vi "Measure Line Distance (SubVI).vi"(9 "Input Valid?":bool=TRUE, 10 "X1 Y1":u32, 11 "X2 Y2":u32) -> (2 "Output Valid?":bool, 3 "Distance":u16)   [LabVIEW 2015]
uses:
  <vilib>/rvi/FXPMathLib/FxpSqrt/subVIs/nifxpmath_Sqrt_SimConfig.ctl
  <vilib>/fxp/LVFixedPointOverflowPolicyTypeDef.ctl
  <vilib>/rvi/FXPMathLib/FxpSqrt/simVIs/DllSqrtTemp_sub.vi
  <vilib>/rvi/FXPMathLib/FxpSub/XNode/nifxpmath_Sub.xnode
  <vilib>/rvi/FXPMathLib/FxpMul/XNode/nifxpmath_Multiplier.xnode
  <vilib>/rvi/FXPMathLib/FxpAdd/XNode/nifxpmath_Add.xnode
  <vilib>/rvi/FXPMathLib/FxpSqrt/XNode/nifxpmath_Sqrt.xnode
  <vilib>/rvi/FXPMathLib/sim/FxpSim.dll
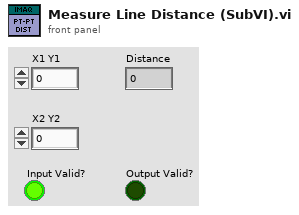
[diagram p1: front panel]
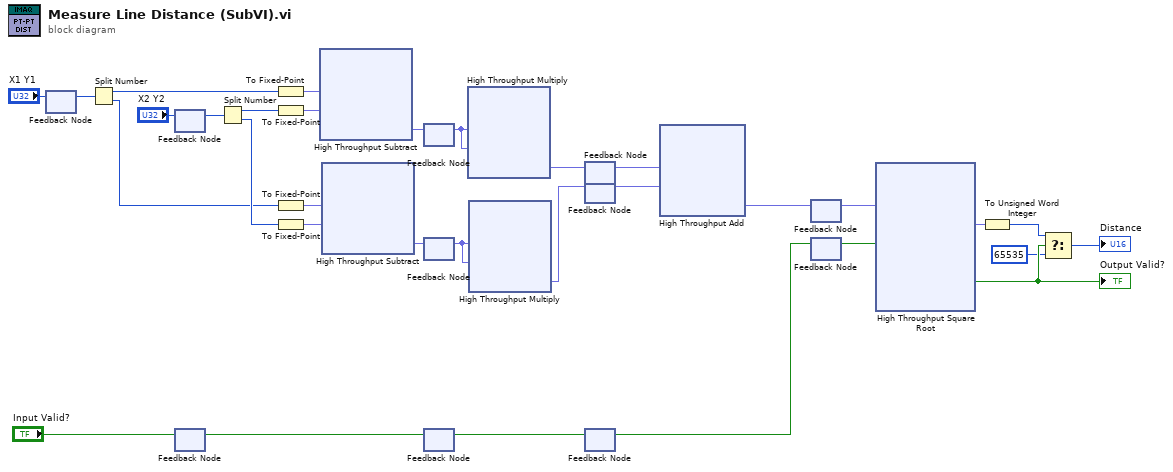
[diagram p0: block diagram]
diagram:
  n1 = feedback-in #1("X1 Y1") -> ()
  n2 = feedback #1() -> (w11:u32)  [unwired: 1 in]
  n3 = Split Number(x=w11) -> (hi(x)=w28:u16, lo(x)=w29:u16)
  n4 = feedback-in #2("X2 Y2") -> ()
  n5 = feedback #2() -> (w10:u32)  [unwired: 1 in]
  n6 = feedback-in #3("Input Valid?") -> ()
  n7 = feedback #3() -> (w9:bool)  [unwired: 1 in]
  n8 = Split Number(x=w10) -> (hi(x)=w31:u16, lo(x)=w32:u16)
  n9 = To Fixed-Point(number=w28) -> (fixed-point=w17:fxp<+/-,16,16>)  [unwired: 1 in]
  n10 = To Fixed-Point(number=w31) -> (fixed-point=w18:fxp<+/-,16,16>)  [unwired: 1 in]
  n11 = To Fixed-Point(number=w29) -> (fixed-point=w20:fxp<+/-,16,16>)  [unwired: 1 in]
  n12 = To Fixed-Point(number=w32) -> (fixed-point=w19:fxp<+/-,16,16>)  [unwired: 1 in]
  n13 = xnode "High Throughput Subtract"("x"=w17, "y"=w18) -> ("x-y"=w21:fxp<+/-,17,17>)
  n14 = xnode "High Throughput Subtract"("x"=w20, "y"=w19) -> ("x-y"=w22:fxp<+/-,17,17>)
  n15 = feedback-in #4(w21) -> ()
  n16 = feedback #4() -> (w8:fxp<+/-,17,17>)  [unwired: 1 in]
  n17 = feedback-in #5(w22) -> ()
  n18 = feedback #5() -> (w7:fxp<+/-,17,17>)  [unwired: 1 in]
  n19 = feedback-in #6(w9) -> ()
  n20 = feedback #6() -> (w6:bool)  [unwired: 1 in]
  n21 = xnode ("High Throughput Multiply")("x"=w8, "y"=w8) -> ("x*y"=w23:fxp<+,32,32>)
  n22 = xnode ("High Throughput Multiply")("x"=w7, "y"=w7) -> ("x*y"=w24:fxp<+,32,32>)
  n23 = feedback-in #7(w23) -> ()
  n24 = feedback #7() -> (w5:fxp<+,32,32>)  [unwired: 1 in]
  n25 = feedback-in #8(w24) -> ()
  n26 = feedback #8() -> (w4:fxp<+,32,32>)  [unwired: 1 in]
  n27 = feedback-in #9(w6) -> ()
  n28 = feedback #9() -> (w3:bool)  [unwired: 1 in]
  n29 = xnode ("High Throughput Add")("x"=w5, "y"=w4) -> ("x+y"=w25:fxp<+,32,32>)
  n30 = feedback-in #10(w25) -> ()
  n31 = feedback #10() -> (w2:fxp<+,32,32>)  [unwired: 1 in]
  n32 = feedback-in #11(w3) -> ()
  n33 = feedback #11() -> (w1:bool)  [unwired: 1 in]
  n34 = xnode "High Throughput Square Root"("x"=w2, "input valid"=w1) -> ("sqrt(x)"=w26:fxp<+,16,16>, "output valid"=w15:bool)  [unwired: 1 in, 1 out]
  "Output Valid?" <- w15
  n35 = To Unsigned Word Integer(number=w26) -> (unsigned 16bit integer=w14:u16)
  n36 = Select(t=w14, s=w15, f=u16 65535) -> (s? t:f=→"Distance":u16)
